vi "Check Parameters.vi"(0 "FM Sweep in":refnum<class "FM Sweep.lvclass">, 9 "Fs (Hz)":dbl, 11 "error in (no error)":errorcluster) -> (4 "FM Sweep out":refnum<class "FM Sweep.lvclass">, 15 "error out":errorcluster)   [LabVIEW 2015, in "FM Sweep.lvclass"]
uses:
  FM Sweep.lvclass
  FM Sweep.lvclass/FM Sweep.ctl
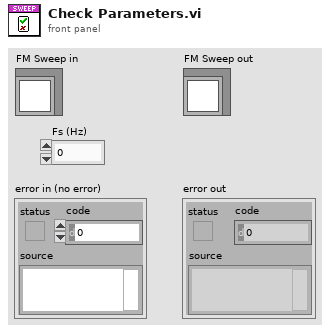
[diagram p1: front panel]
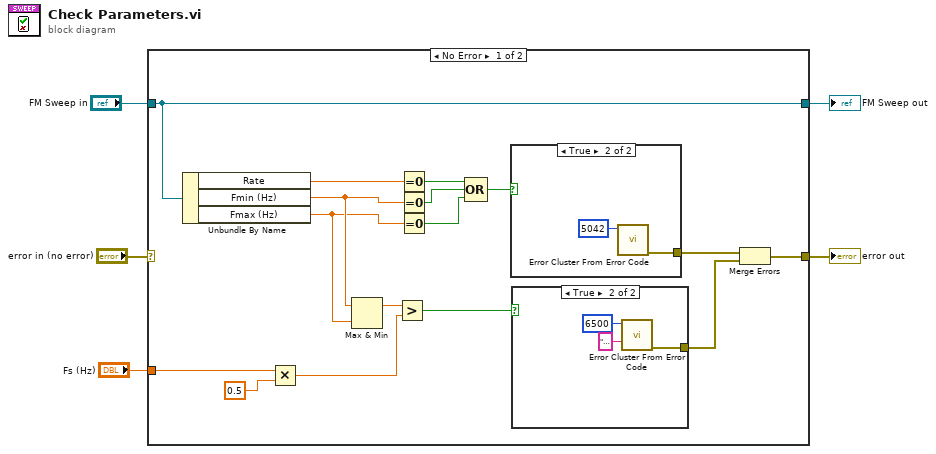
[diagram p0: block diagram]
diagram:
  n1 = case shown="No Error" "error in (no error)" {
    selector: "error in (no error)" -> [_ w28]
    tunnel: [w7 w28] -> w4
    tunnel: [w17 w27] -> w2
    tunnel: "FM Sweep in" -> [w17 w27]
    tunnel: "Fs (Hz)" -> [w11 _]
    frame No Error {
      n2 = Unbundle By Name(w17) -> ("Rate"=w15:dbl, "Fmin (Hz)"=w14:dbl, "Fmax (Hz)"=w13:dbl)
      n3 = Multiply(x=w11, y=0.5) -> (x*y=w9:dbl)
      n4 = Max & Min(x=w14, y=w13) -> (max(x,y)=w12:dbl)  [unwired: 1 out]
      n5 = Greater?(x=w12, y=w9) -> (0:w8:bool)
      n6 = Equal To 0?(x=w15) -> (x = 0?=w18:bool)
      n7 = Equal To 0?(x=w14) -> (x = 0?=w19:bool)
      n8 = Equal To 0?(x=w13) -> (x = 0?=w20:bool)
      n9 = Compound Arithmetic op=OR(w18, w19, w20) -> (w21:bool)
      n10 = case shown="True" w21 {
        tunnel: [_ w26] -> w16
        frame False {
        }
        frame True {
          n11 = call <vilib>:"Error Cluster From Error Code.vi"("error code (0)"=5042) -> ("error out"=w26:errorcluster)  [unwired: 8 in]
        }
      }
      n12 = case shown="True" w8 {
        tunnel: [_ w23] -> w6
        frame False {
        }
        frame True {
          n13 = call <vilib>:"Error Cluster From Error Code.vi"("error message (\"\")"="FM Sweep: Fmax exceeds the Nyquist frequency. Increase the sampling rate or decrease Fmax." ("error message (\"\")"), "error code (0)"=6500) -> ("error out"=w23:errorcluster)  [unwired: 7 in]
        }
      }
      n14 = Merge Errors(w16, w6) -> (w7:errorcluster)
    }
    frame Error {
    }
  }
  "error out" <- w4
  "FM Sweep out" <- w2
